vi "Example_DataRecording.vi"() -> ()   [LabVIEW 2017, in "maxonEPOS.lvlib"]
doc: "Example how to configure and use the data recording functions. Before starts this example the device must be tuned and the parameter settings must be correct.\nThe example shows:\n - how to initialise and close an interface (e.g. RS232)\n - configuration of the data recorder\n - start of a relative positioning\n - show the recorded data (position, velocity and current)"
uses:
  maxonEPOS.lvlib
panel:
  out "Current  Graph":i32[](graph)
  out "Velocity Graph":i32[](graph)
  out "Position  Graph":i32[](graph)
  in  "timeout":u32=1000
  in  "relative position":i32=100
  in  "position profile":T1={"profileVelocity"=1000, "profileAcceleration"=10000, "profileDeceleration"=10000}
  in  "nodeId":u16=1
  in  "communication settings in":T2={"deviceName"="EPOS2", "protocolStackName"="MAXON SERIAL V2", "interfaceName"="USB", "portName"="USB0", "baudrate"=1000000, "timeout"=500}
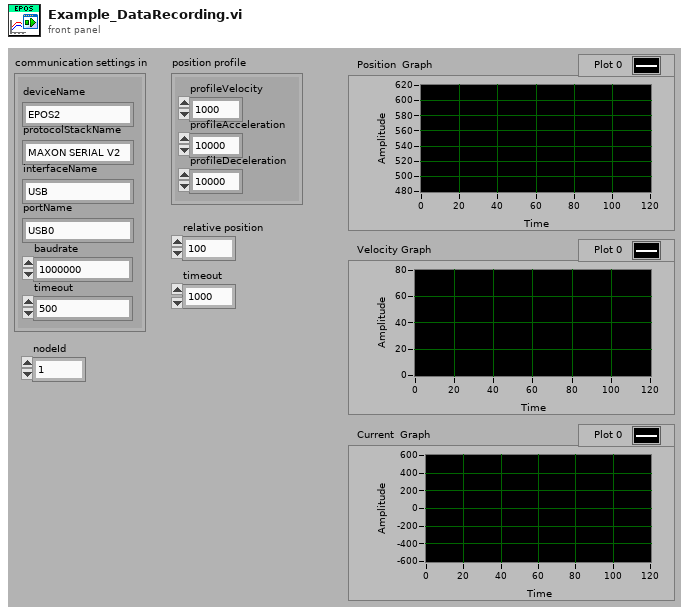
[diagram p1: front panel]
types:
  T1 = cluster{"profileVelocity":u32, "profileAcceleration":u32, "profileDeceleration":u32}
  T2 = cluster{"deviceName":string, "protocolStackName":string, "interfaceName":string, "portName":string, "baudrate":u32, "timeout":u32}
  T3 = cluster{"samplingPeriod":u16, "nbOfPrecedingSamples":u16}
  T4 = cluster{"recorded object 1":cluster{"objectIndex":u16, "objectSubIndex":u8, "objectSize":u8}, "recorded object 2":cluster{"objectIndex":u16, "objectSubIndex":u8, "objectSize":u8}, "recorded object 3":cluster{"objectIndex":u16, "objectSubIndex":u8, "objectSize":u8}, "recorded object 4":cluster{"objectIndex":u16, "objectSubIndex":u8, "objectSize":u8}}
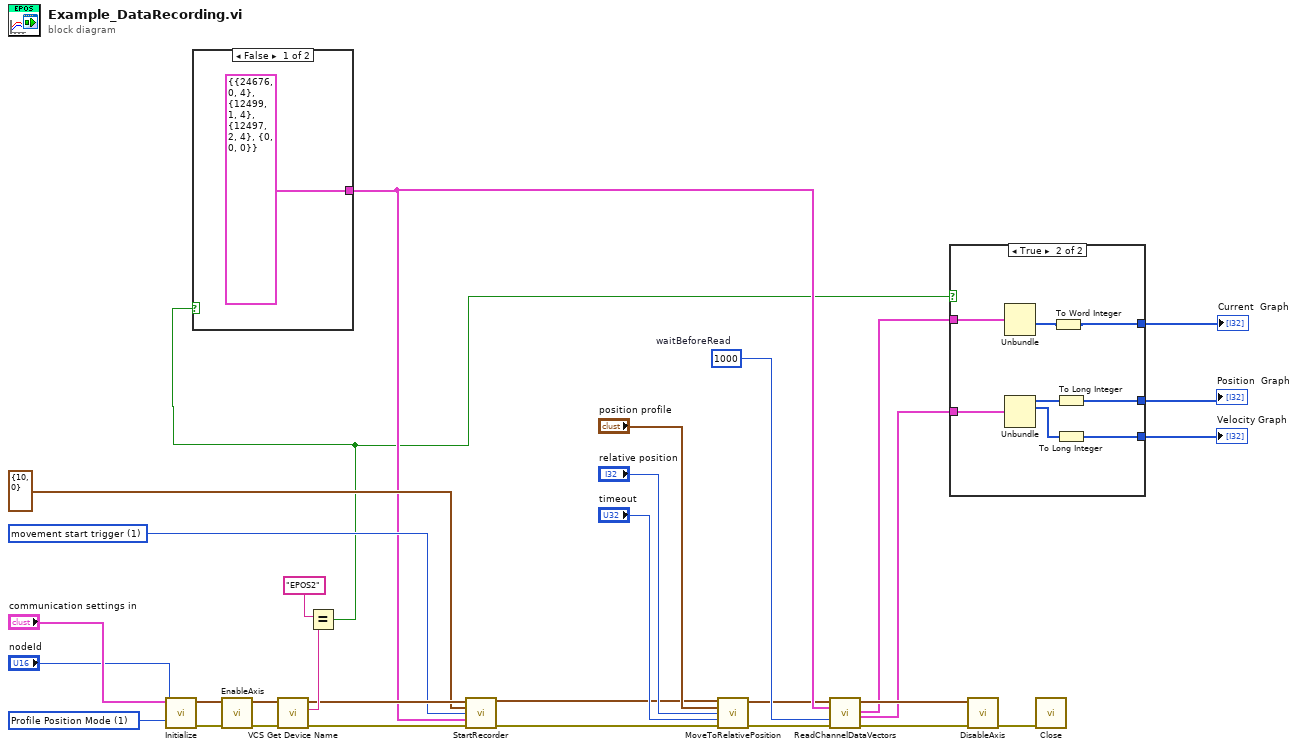
[diagram p0: block diagram]
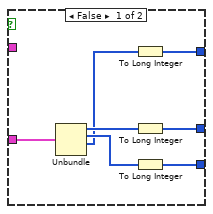
[diagram p2: hidden frame]
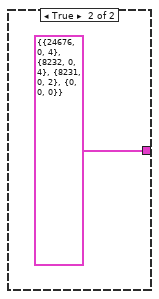
[diagram p3: hidden frame]
diagram:
  w13 = u32 1000  # waitBeforeRead
  w16 = u8 1 items=["movement start trigger"=1, "error trigger"=2, "digital input trigger"=4, "movement end trigger"=8] ("trigger type")
  w30 = i8 1 items=["Profile Position Mode"=1, "Profile Velocity Mode"=3, "Homing Mode"=6, "Interpolated Position Mode"=7, "Position Mode"=-1, "Velocity Mode"=-2, "Current Mode"=-3, "Master Encoder Mode"=-5, "Step Direction Mode"=-6] ("modes of operations")
  n1 = call "Initialize.vi"("modes of operations"=w30, "nodeId"="nodeId", "communication settings in"="communication settings in") -> ("error out"=w28:errorcluster, "axis out"=w27:cluster{"keyHandle":u32, "nodeId":u16})  [unwired: 7 in]
  n2 = call "EnableAxis.vi"("error in (no error)"=w28, "axis in"=w27) -> ("error out"=w21:errorcluster, "axis out"=w22:cluster{"keyHandle":u32, "nodeId":u16})  [unwired: 4 in]
  n3 = call "VCS Get Device Name.vi"("error in (no error)"=w21, "axis in"=w22) -> ("error out"=w15:errorcluster, "deviceName"=w20:string, "axis out"=w18:cluster{"keyHandle":u32, "nodeId":u16})  [unwired: 7 in]
  n4 = Equal?(x=w20, y="EPOS2" ("x")) -> (x = y?=w5:bool)
  n5 = case shown="False" w5 {
    tunnel: [T4 {"recorded object 1"={"objectIndex"=24676, "objectSubIndex"=0, "objectSize"=4}, "recorded object 2"={"objectIndex"=12499, "objectSubIndex"=1, "objectSize"=4}, "recorded object 3"={"objectIndex"=12497, "objectSubIndex"=2, "objectSize"=4}, "recorded object 4"={"objectIndex"=0, "objectSubIndex"=0, "objectSize"=0}} ("recorded objects") T4 {"recorded object 1"={"objectIndex"=24676, "objectSubIndex"=0, "objectSize"=4}, "recorded object 2"={"objectIndex"=8232, "objectSubIndex"=0, "objectSize"=4}, "recorded object 3"={"objectIndex"=8231, "objectSubIndex"=0, "objectSize"=2}, "recorded object 4"={"objectIndex"=0, "objectSubIndex"=0, "objectSize"=0}} ("recorded objects")] -> w14
    frame False {
    }
    frame True {
    }
  }
  n6 = call "StartRecorder.vi"("axis in"=w18, "parameter"=T3 {"samplingPeriod"=10, "nbOfPrecedingSamples"=0}, "trigger type"=w16, "recorded objects"=w14, "error in (no error)"=w15) -> ("axis out"=w12:cluster{"keyHandle":u32, "nodeId":u16}, "error out"=w11:errorcluster)  [unwired: 9 in]
  n7 = call "MoveToRelativePosition.vi"("axis in"=w12, "position profile"="position profile", "relative position"="relative position", "timeout"="timeout", "error in (no error)"=w11) -> ("axis out"=w7:cluster{"keyHandle":u32, "nodeId":u16}, "error out"=w10:errorcluster)  [unwired: 9 in]
  n8 = call "ReadChannelDataVectors.vi"("axis in"=w7, "recorded objects"=w14, "waitBeforeRead"=w13, "error in (no error)"=w10) -> ("axis out"=w8:cluster{"keyHandle":u32, "nodeId":u16}, "U16 data vectors"=w6:cluster{u16[], u16[], u16[], u16[]}, "U32 data vectors"=w4:cluster{u32[], u32[], u32[], u32[]}, "error out"=w9:errorcluster)  [unwired: 7 in, 1 out]
  n9 = case shown="True" w5 {
    tunnel: w6 -> [_ w48]
    tunnel: w4 -> [w38 w45]
    tunnel: [w34 w42] -> w1
    tunnel: [w37 w44] -> w3
    tunnel: [w36 w43] -> w2
    frame False {
      n10 = Unbundle(w38) -> (w40:u32[], w39:u32[], w35:u32[])  [unwired: 1 out]
      n11 = To Long Integer(number=w35) -> (32bit integer=w34:i32[])
      n12 = To Long Integer(number=w40) -> (32bit integer=w37:i32[])
      n13 = To Long Integer(number=w39) -> (32bit integer=w36:i32[])
    }
    frame True {
      n14 = Unbundle(w48) -> (w41:u16[])  [unwired: 3 out]
      n15 = Unbundle(w45) -> (w46:u32[], w47:u32[])  [unwired: 2 out]
      n16 = To Word Integer(number=w41) -> (16bit integer=w42:i16[])
      n17 = To Long Integer(number=w46) -> (32bit integer=w44:i32[])
      n18 = To Long Integer(number=w47) -> (32bit integer=w43:i32[])
    }
  }
  "Position  Graph" <- w3
  "Velocity Graph" <- w2
  "Current  Graph" <- w1
  n19 = call "DisableAxis.vi"("error in (no error)"=w9, "axis in"=w8) -> ("error out"=w23:errorcluster)  [unwired: 4 in, 1 out]
  n20 = call "Close.vi"("error in (no error)"=w23) -> ()  [unwired: 10 in, 1 out]
